vi "State_Machine.vi"(8 "error in (no error)":errorcluster caption="entrée d'erreur (pas d'erreur)", 11 "Get_Voltage en entrée":refnum<class "Zigbee_Stop_Permit_Join.lvclass">) -> (0 "error out":errorcluster caption="sortie d'erreur", 2 "Json_String":string, 3 "Get_Voltage en sortie":refnum<class "Zigbee_Stop_Permit_Join.lvclass">)   [LabVIEW 2020, in "Library Test.lvlib" / "Zigbee_Stop_Permit_Join.lvclass"]
uses:
  Zigbee_Stop_Permit_Join.lvclass
  C:/Users/ngarcin/OneDrive - Altyor/Standard TB/Class/Test/Zigbee_Send_Command_UART/Zigbee_Send_Command_UART.lvclass
  Zigbee_Send_Command_UART/Zigbee_Send_Command_UART.lvclass
  Zigbee_Stop_Permit_Join.lvclass/Zigbee_Stop_Permit_Join.ctl
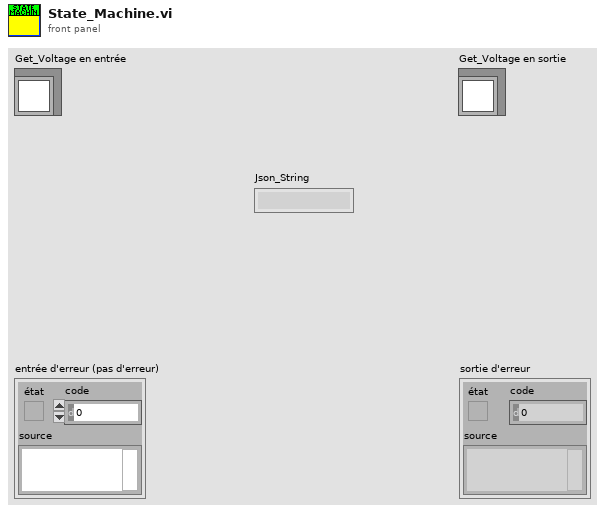
[diagram p1: front panel]
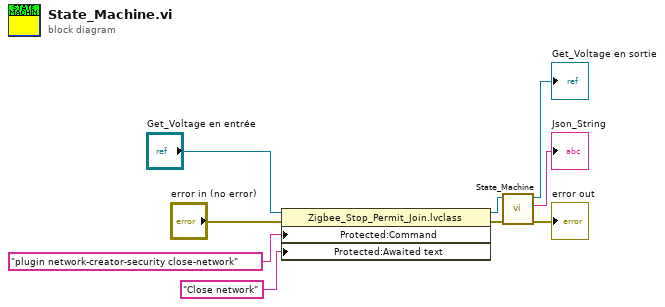
[diagram p0: block diagram]
diagram:
  n1 = property class="Zigbee_Stop_Permit_Join.lvclass"(reference="Get_Voltage en entrée", error in="error in (no error)", "Protected:Command"="plugin network-creator-security close-network" ("Command"), "Protected:Awaited text"="Close network" ("Command")) -> (reference out=w6:refnum<class "Zigbee_Stop_Permit_Join.lvclass">, error out=w5:errorcluster)
  n2 = call-parent "State_Machine.vi"("error in (no error)"=w5, "Send_Frame en entrée"=w6) -> ("error out"=→"error out":errorcluster, "Json_String"=→"Json_String":string, "Send_Frame en sortie"=→"Get_Voltage en sortie":refnum<class "Zigbee_Stop_Permit_Join.lvclass">)  [unwired: 7 in]
